vi "Create.vi"(8 "error in (no error)":errorcluster, 11 "JKI SMO in":refnum<class "JKI SMO.lvclass">) -> (0 "error out":errorcluster, 3 "JKI SMO out":refnum<class "JKI SMO.lvclass">)   [LabVIEW 2013, in "JKI SMO.lvclass"]
doc: "Constructor\n\nNote 01: This method is overridable by descendant\nNote 02: When overridden, Call Parent Method is required\n\n---------------------------------------------------------------\nJKI State Machine Objects™\nhttp://jki.net/state-machine-objects/\nCopyright (C) 2005-2015, JKI <info@jki.net>\nALL RIGHTS RESERVED"
uses:
  JKI SMO.lvclass
  Typedefs/StopProcessEventData--Cluster.ctl
  Typedefs/AbortProcessEventData--Cluster.ctl
  JKI SMO.lvclass/JKI SMO.ctl
panel:
  # "For instructions on how to use the JKI State Machine Objects, examples and video tutorials, visit:\nhttp://jki.net/state-machine-objects/\n\nJKI State Machine Objects™\nhttp://jki.net/state-machine-objects/\nCopyright (C) 2005-2015, JKI <info@jki.net>\nALL RIGHTS RESERVED"
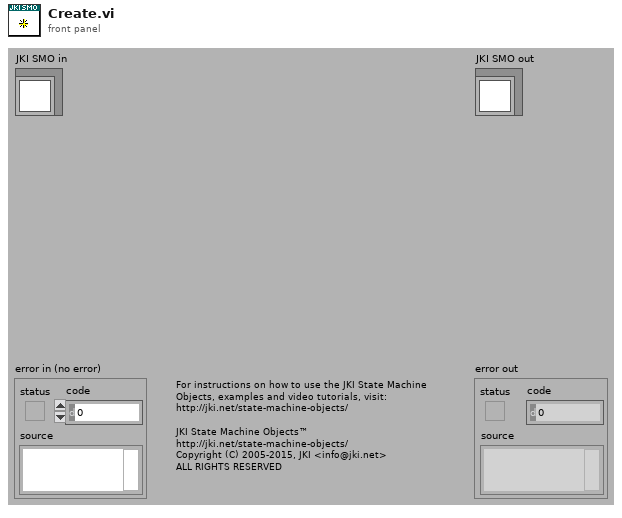
[diagram p1: front panel]
types:
  T1 = typedef "JKI SMO.lvclass/AbortProcessEventData--Cluster.ctl" = cluster{"Time Stamp":timestamp}
  T2 = typedef "JKI SMO.lvclass/StopProcessEventData--Cluster.ctl" = cluster{"Time Stamp":timestamp}
  T3 = typedef "JKI SMO.lvclass/PrivateData--Cluster.ctl" = cluster{"Processes Clone VI Ref [ ]":refnum<vi>[], "Processes Clone Name [ ]":string[], "Process Sync RendezVous":T4, "Protected Events":T5, "Registered Process [ ]":T6[]}
  T4 = typedef "Rendezvous RefNum" = refnum<k1>
  T5 = typedef "JKI SMO.lvclass/ProtectedEvents--Cluster.ctl" = cluster{"StopProcesses":refnum<user-event>, "AbortProcesses":refnum<user-event>}
  T6 = typedef "JKI SMO.lvclass/RegisteredProcessData--Cluster.ctl" = cluster{"Name":string, "Static VI Ref":refnum<vi>}
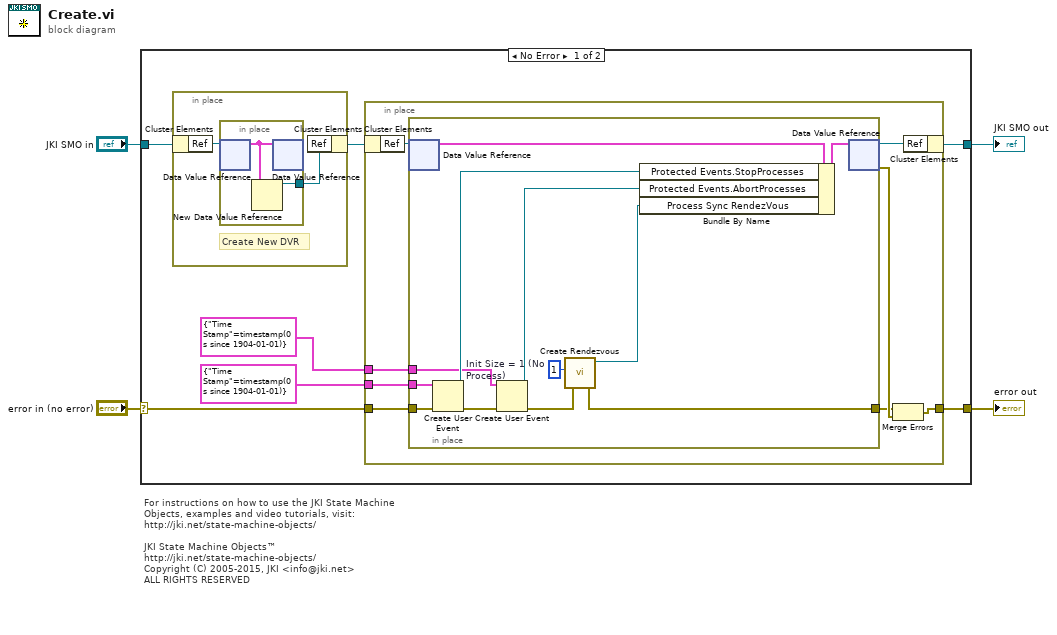
[diagram p0: block diagram]
diagram:
  # "For instructions on how to use the JKI State Machine Objects, examples and video tutorials, visit:\nhttp://jki.net/state-machine-objects/\n\nJKI State Machine Objects™\nhttp://jki.net/state-machine-objects/\nCopyright (C) 2005-2015, JKI <info@jki.net>\nALL RIGHTS RESERVED"
  n1 = case shown="No Error" "error in (no error)" {
    selector: "error in (no error)" -> [w9 w37]
    tunnel: [w6 w37] -> w3
    tunnel: [w7 w36] -> w1
    tunnel: "JKI SMO in" -> [w11 w36]
    frame No Error {
      n2 = in-place {
        # "Create New DVR"
        n3 = in-place-cluster #1(w11) -> ("Ref"=w33:refnum<data-value>)
        n4 = in-place {
          in-place-border: [w35] -> w32
          n5 = in-place-dvr #2(w33) -> (w34:T3)  [unwired: 1 out]
          n6 = New Data Value Reference(data value=w34) -> (data value reference=w35:refnum<data-value>)  [unwired: 1 in, 1 out]
          n7 = in-place-dvr #2(w34) -> ()  [unwired: 2 out]
        }
        n8 = in-place-cluster #1("Ref"=w32) -> (w10:refnum<class "JKI SMO.lvclass">)
      }
      n9 = in-place {
        in-place-border: w9 -> [w17]
        in-place-border: T2 {"Time Stamp"=timestamp(0 s since 1904-01-01)} ("Stop Processes Event Data") -> [w16]
        in-place-border: [w14] -> w6
        in-place-border: T1 {"Time Stamp"=timestamp(0 s since 1904-01-01)} ("Abort Processes Event Data") -> [w12]
        n10 = in-place-cluster #3(w10) -> ("Ref"=w19:refnum<data-value>)
        n11 = in-place {
          in-place-border: w17 -> [w30]
          in-place-border: w16 -> [w29]
          in-place-border: [w26] -> w13
          in-place-border: w12 -> [w21]
          w24 = 1  # Init Size = 1 (No Process)
          n12 = in-place-dvr #4(w19) -> (w31:T3)  [unwired: 1 out]
          n13 = Create User Event(user event datatype=w29, error in=w30) -> (user event=w27:refnum<user-event>, error out=w23:errorcluster)
          n14 = Create User Event(user event datatype=w21, error in=w23) -> (user event=w20:refnum<user-event>, error out=w22:errorcluster)
          n15 = call <vilib>:"Create Rendezvous.vi"("error in (no error)"=w22, "size (2)"=w24) -> ("error out"=w26:errorcluster, "rendezvous"=w25:T4)  [unwired: 3 in, 1 out]
          n16 = Bundle By Name(cluster=w31, "Protected Events.StopProcesses"=w27, "Protected Events.AbortProcesses"=w20, "Process Sync RendezVous"=w25) -> (w28:T3)
          n17 = in-place-dvr #4(w28) -> (w18:refnum<data-value>, w15:errorcluster)
        }
        n18 = Merge Errors(w13, w15) -> (w14:errorcluster)
        n19 = in-place-cluster #3("Ref"=w18) -> (w7:refnum<class "JKI SMO.lvclass">)
      }
    }
    frame Error {
    }
  }
  "error out" <- w3
  "JKI SMO out" <- w1
